vi "Add Argument.vi"(8 "error in (no error)":errorcluster, 9 "Value":variant, 10 "Name":string, 11 "Arguments in":refnum<class "Arguments.lvclass">) -> (0 "error out":errorcluster, 3 "Arguments out":refnum<class "Arguments.lvclass">)   [LabVIEW 2020, in "HTTP Server.lvlib" / "Arguments.lvclass"]
uses:
  Arguments.lvclass
  Arguments.lvclass/Arguments.ctl
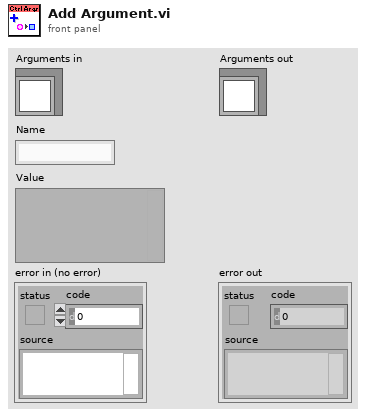
[diagram p1: front panel]
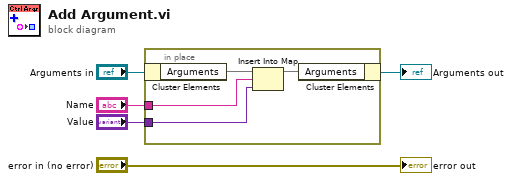
[diagram p0: block diagram]
diagram:
  n1 = in-place {
    in-place-border: "Name" -> [w8]
    in-place-border: "Value" -> [w7]
    n2 = in-place-cluster #1("Arguments in") -> ("Arguments"=w9:map{string, variant})
    n3 = Insert Into Map(map in=w9, key=w8, value=w7) -> (map out=w6:map{string, variant})  [unwired: 2 out]
    n4 = in-place-cluster #1("Arguments"=w6) -> (→"Arguments out":refnum<class "Arguments.lvclass">)
  }
  "error out" <- "error in (no error)"
